vi "Configure Coupling.vi"(6 "Enable Coupling (T: Enable)":bool=TRUE, 7 "Deviation (0)":dbl, 8 "error in (no error)":errorcluster, 9 "Base Channel (1: Channel 1)":i32(ring)=1 items=["Channel 1"=1, "Channel 2"=2], 10 "Action Type (0: Set Amplitude Coupling)":i32(ring) items=["Set Amplitude Coupling", "Set Frequency Coupling", "Set Phase Coupling", "Set Base Channel"], 11 "VISA resource name":refnum<visa-resource-name>) -> (0 "error out":errorcluster, 3 "VISA resource name out":refnum<visa-resource-name>)   [LabVIEW 2015, in "RIGOL DG4000 Series.lvlib"]
doc: "Configures the base channel, frequency coupling, phase coupling and amplitude coupling settings."
uses:
  <instrlib>/RIGOL DG4000 Series/RIGOL DG4000 Series.lvlib
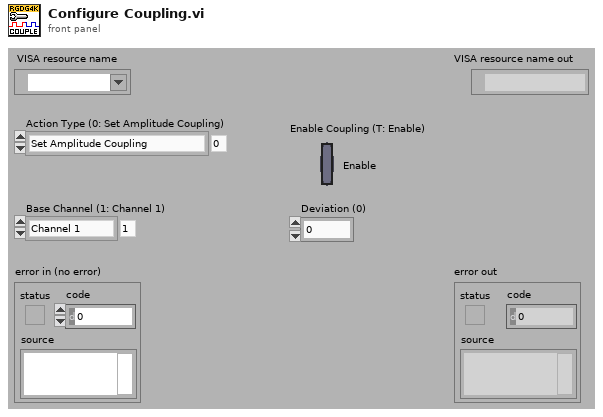
[diagram p1: front panel]
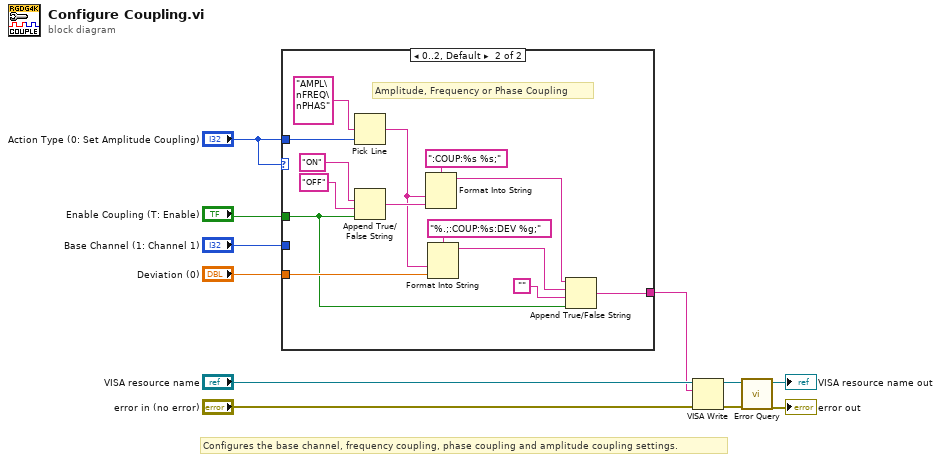
[diagram p0: block diagram]
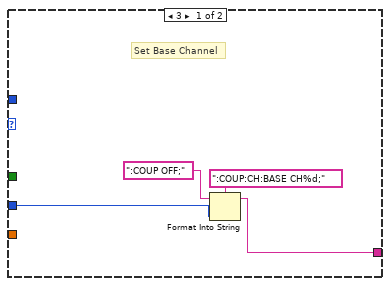
[diagram p2: hidden frame]
diagram:
  # "Configures the base channel, frequency coupling, phase coupling and amplitude coupling settings."
  n1 = case shown="0..2, Default" "Action Type (0: Set Amplitude Coupling)" {
    tunnel: "Action Type (0: Set Amplitude Coupling)" -> [_ w28]
    tunnel: "Deviation (0)" -> [_ w26]
    tunnel: "Enable Coupling (T: Enable)" -> [_ w17]
    tunnel: "Base Channel (1: Channel 1)" -> [w14 _]
    tunnel: [w13 w16] -> w1
    frame 3 {
      # "Set Base Channel"
      n2 = Format Into String(format string=":COUP:CH:BASE CH%d;", initial string=":COUP OFF;", w14) -> (resulting string=w13:string)  [unwired: 1 in, 1 out]
    }
    frame 0..2, Default {
      # "Amplitude, Frequency or Phase Coupling"
      n3 = Pick Line(multi-line string="AMPL\nFREQ\nPHAS", line index=w28) -> (output string=w21:string)  [unwired: 1 out]
      n4 = Append True/False String(1:w17, 2:"OFF", 3:"ON") -> (0:w22:string)  [unwired: 1 out]
      n5 = Format Into String(format string=":COUP:%s %s;", w21, w22) -> (resulting string=w20:string)  [unwired: 2 in, 1 out]
      n6 = Format Into String(format string="%.;:COUP:%s:DEV %g;", w21, w26) -> (resulting string=w19:string)  [unwired: 2 in, 1 out]
      n7 = Append True/False String(1:w17, 2:"", 3:w19, 4:w20) -> (0:w16:string)
    }
  }
  n8 = VISA Write(VISA resource name="VISA resource name", write buffer=w1, error in (no error)="error in (no error)") -> (VISA resource name out=w7:refnum<visa-resource-name>, error out=w6:errorcluster)  [unwired: 1 out]
  n9 = call <instrlib>:"Error Query.vi"("error in (no error)"=w6, "VISA resource name"=w7) -> ("error out"=→"error out":errorcluster, "VISA resource name out"=→"VISA resource name out":refnum<visa-resource-name>)  [unwired: 8 out]
